vi "NCDC Weather API Demo.vi"() -> ()   [LabVIEW 2020]
uses:
  Dynamic Combobox/Dynamic Combobox/Options.ctl
  NCDC Weather/NCDC Weather.lvclass
  C:/dev/NI/Dynamic Combobox/Dynamic Combobox/Dynamic Values/Dynamic Values.lvclass
  Dynamic Combobox/Dynamic Combobox/Dynamic Combobox.lvclass
  <vilib>/httpClient/LabVIEWHTTPClient.lvlib
panel:
  out "headers":string
  out "body":string
  in  "Location":string(combo)
  in  "NCDC Token":string
  # "To use this demo, register for an API token at https://www.ncdc.noaa.gov/cdo-web/token\n\nOnce you have received this token enter it in the NCDC Token input and then you can run the VI."
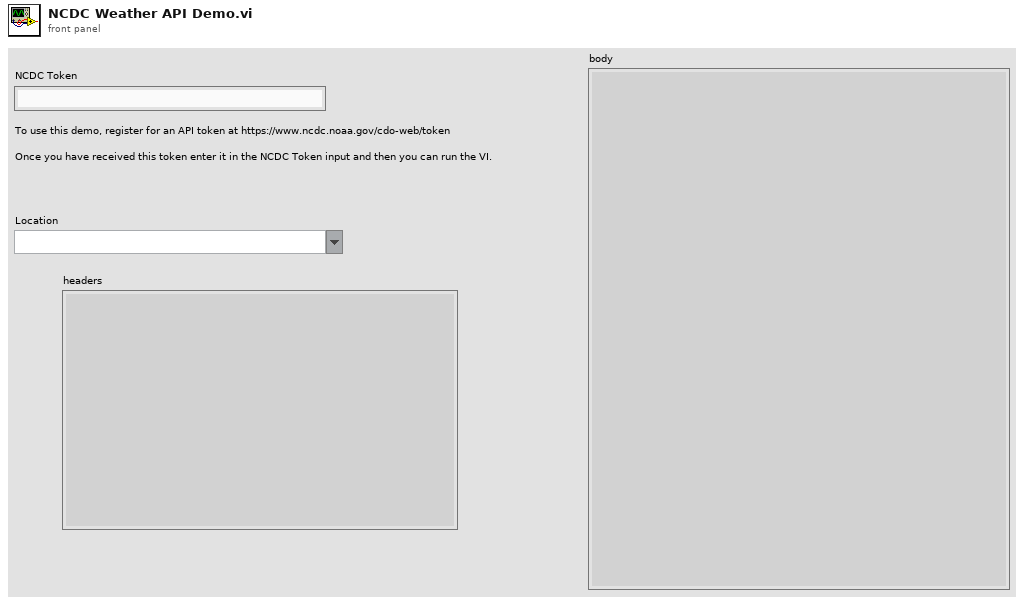
[diagram p1: front panel]
types:
  T1 = typedef "Dynamic Combobox.lvlib/Dynamic Combobox.lvclass/Options.ctl" = cluster{"Browse Entry":bool, "Refresh Entry":bool}
  T2 = typedef "Dynamic Combobox.lvlib/Dynamic Combobox.lvclass/Dynamic Combobox Events.ctl" = cluster{"Selection":refnum<user-event>, "Error":refnum<user-event>}
  T3 = typedef "LabVIEWHTTPClient.lvlib/ClientHandle.ctl" = refnum<k1>
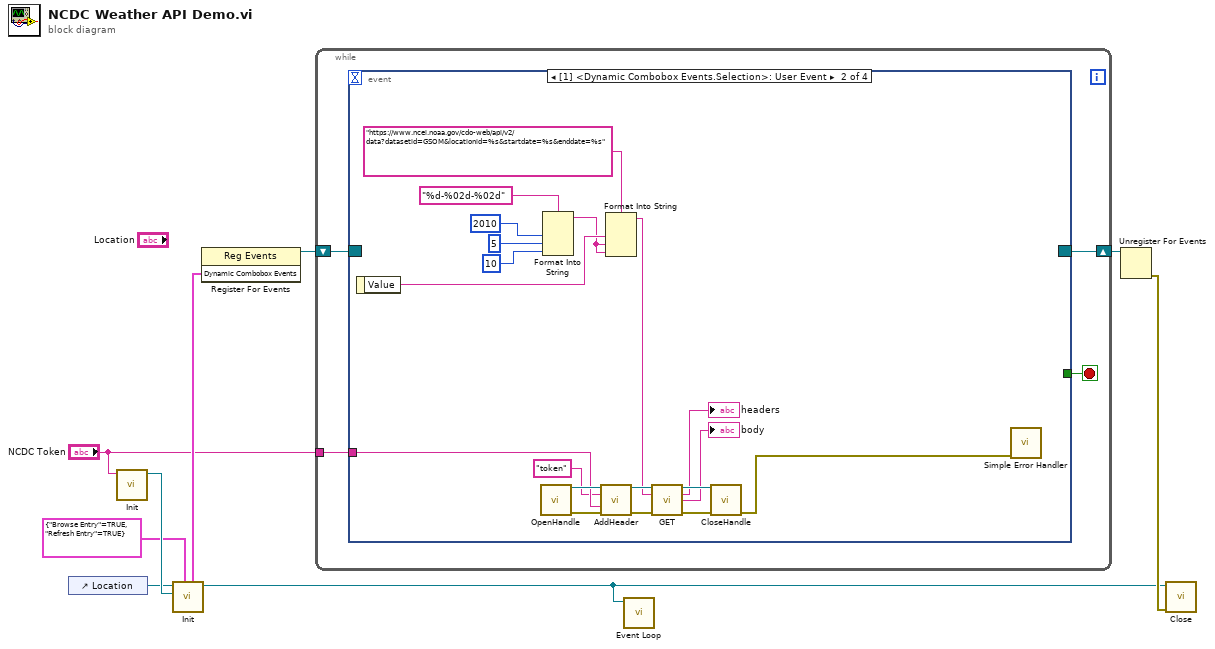
[diagram p0: block diagram]
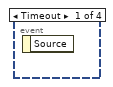
[diagram p2: hidden frame]
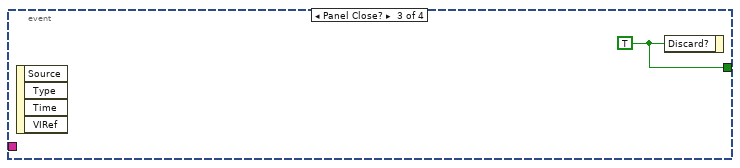
[diagram p3: hidden frame]
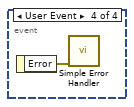
[diagram p4: hidden frame]
diagram:
  n1 = control-ref of="Location"() -> (w7:refnum<vi>)
  n2 = call "Init.vi"("Token"="NCDC Token") -> ("NCDC Weather out"=w8:refnum<class "NCDC Weather.lvclass">)  [unwired: 9 in, 1 out]
  n3 = call "Init.vi"("Options (None)"=T1 {"Browse Entry"=TRUE, "Refresh Entry"=TRUE}, "Dynamic Values"=w8, "Combobox"=w7) -> ("Dynamic Combobox out"=w1:refnum<class "Dynamic Combobox.lvclass">, "Dynamic Combobox Events"=w5:T2)  [unwired: 6 in, 1 out]
  n4 = register-events(w5) -> (reference out=w3:refnum<event-registration>)  [unwired: 2 in, 1 out]
  n5 = while {
    tunnel: "NCDC Token" -> [w11]
    shift-right: [w12] -> w2
    shift-left: w3 -> [w13]
    stop <- w10 stop-if-true
    n6 = event shown="[1] <Dynamic Combobox Events.Selection>: User Event" {
      selector: w13 -> [_ _ _ _]
      dyn-events: [_ _ _ _] -> w12
      timeout: _ -> [_ _ _ _]
      tunnel: w11 -> [_ w30 _ _]
      tunnel: [_ _ w33 _] -> w10
      event Timeout {
        n7 = event-data() -> ()  [unwired: 1 in, 1 out]
      }
      event User Event {
        n8 = event-data() -> ("Value"=w22:string)  [unwired: 1 in]
        n9 = call <vilib>:"OpenHandle.vi"() -> ("client handle out"=w31:T3, "error out"=w32:errorcluster)  [unwired: 14 in]
        n10 = Format Into String(format string="%d-%02d-%02d", 2010 ("input 1"), 5 ("input 1"), 10 ("input 1")) -> (resulting string=w21:string)  [unwired: 2 in, 1 out]
        n11 = call <vilib>:"AddHeader.vi"("client handle"=w31, "header"="token", "value"=w30, "error in (no error)"=w32) -> ("client handle out"=w28:T3, "error out"=w25:errorcluster)  [unwired: 10 in]
        n12 = Format Into String(format string="https://www.ncei.noaa.gov/cdo-web/api/v2/data?datasetid=GSOM&locationid=%s&startdate=%s&enddate=%s", w22, w21, w21) -> (resulting string=w14:string)  [unwired: 2 in, 1 out]
        n13 = call <vilib>:"GET.vi"("client handle"=w28, "url"=w14, "error in (no error)"=w25) -> ("client handle out"=w26:T3, "headers"=→"headers":string, "body"=→"body":string, "error out"=w24:errorcluster)  [unwired: 9 in]
        n14 = call <vilib>:"CloseHandle.vi"("client handle"=w26, "error in (no error)"=w24) -> ("error out"=w19:errorcluster)  [unwired: 13 in]
        n15 = call <vilib>:"Simple Error Handler.vi"("error in (no error)"=w19) -> ()  [unwired: 4 in, 5 out]
      }
      event Panel Close? {
        w33 = TRUE ("Discard?")
        n16 = event-data() -> ()  [unwired: 1 in, 4 out]
        n17 = event-data("Discard?"=w33) -> ()  [unwired: 1 in, 1 out]
      }
      event User Event {
        n18 = event-data() -> ("Error"=w34:errorcluster)  [unwired: 1 in]
        n19 = call <vilib>:"Simple Error Handler.vi"("error in (no error)"=w34) -> ()  [unwired: 4 in, 5 out]
      }
    }
  }
  n20 = call "Event Loop.vi"("Dynamic Combobox in"=w1) -> ()  [unwired: 10 in, 1 out]
  n21 = Unregister For Events(event registration refnum=w2) -> (error out=w9:errorcluster)  [unwired: 1 in]
  n22 = call "Close.vi"("error in (no error)"=w9, "Dynamic Combobox in"=w1) -> ()  [unwired: 9 in, 1 out]
